vi "Get Item From Index.vi"(8 "错误输入":errorcluster, 9 "Index":i32, 11 "Listbox Ref":refnum<vi>) -> (0 "错误输出":errorcluster, 2 "Item":string, 3 "Dup Listbox Ref":refnum<vi>)   [LabVIEW 2012, in "Listbox Tool.lvlib"]
uses:
  Listbox Tool.lvlib
  Property/Set and Get ItemNames.vi
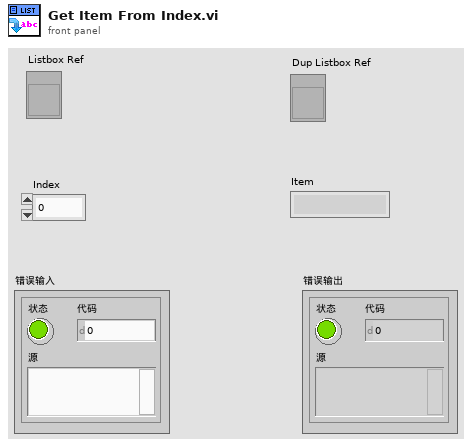
[diagram p1: front panel]
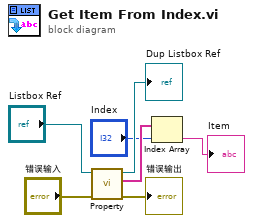
[diagram p0: block diagram]
diagram:
  n1 = call-poly "Property.vi"("错误输入"="错误输入", "Listbox Ref"="Listbox Ref") -> ("错误输出"=→"错误输出":errorcluster, "ItemNames Out"=w5:string[], "Dup Listbox Ref"=→"Dup Listbox Ref":refnum<vi>)  [unwired: 7 in]
  n2 = Index Array(array=w5, index="Index") -> (element=→"Item":string)
